vi "lab3sub.vi"(9 "error in (no error)":errorcluster, 10 "write buffer":string) -> (1 "error out 2":errorcluster, 2 "read buffer":string)   [LabVIEW 2018]
panel:
  out "VISA resource name out 2":refnum<visa-resource-name>
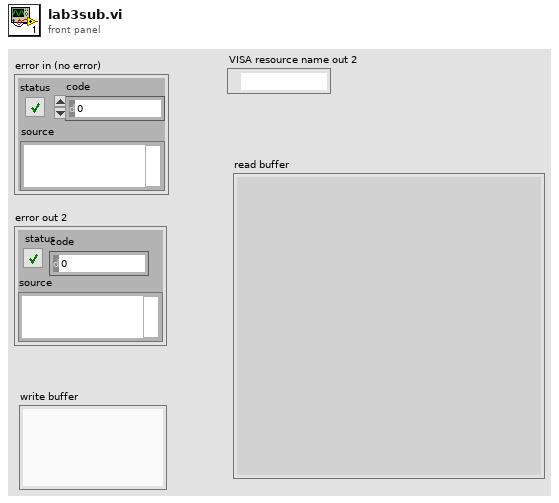
[diagram p1: front panel]
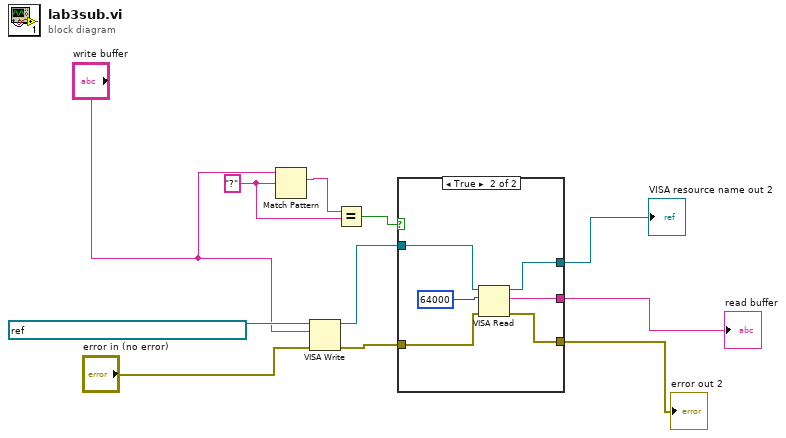
[diagram p0: block diagram]
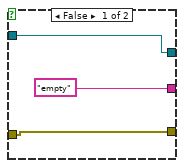
[diagram p2: hidden frame]
diagram:
  w2 = "?" ("regular expression")
  n1 = Match Pattern(string="write buffer", regular expression=w2) -> (match substring=w6:string)  [unwired: 1 in, 3 out]
  n2 = VISA Write(VISA resource name=refnum<visa-resource-name> "USB0::0x0699::0x0368::C040642::INSTR", write buffer="write buffer", error in (no error)="error in (no error)") -> (VISA resource name out=w9:refnum<visa-resource-name>, error out=w8:errorcluster)  [unwired: 1 out]
  n3 = Equal?(x=w6, y=w2) -> (x = y?=w3:bool)
  n4 = case shown="True" w3 {
    tunnel: w9 -> [w13 w19]
    tunnel: w8 -> [w14 w18]
    tunnel: [w13 w17] -> w5
    tunnel: ["empty" w16] -> w1
    tunnel: [w14 w15] -> w4
    frame False {
    }
    frame True {
      n5 = VISA Read(VISA resource name=w19, byte count=64000, error in (no error)=w18) -> (VISA resource name out=w17:refnum<visa-resource-name>, read buffer=w16:string, error out=w15:errorcluster)  [unwired: 1 out]
    }
  }
  "error out 2" <- w4
  "read buffer" <- w1
  "VISA resource name out 2" <- w5
